vi "LVClass_Pupil ctor from dimensions.vi"(0 "Pupil (const)":refnum<class "Pupil.lvclass">, 5 "Dimensions_um":T1, 7 "value":u8=1, 11 "error in (no error)":errorcluster) -> (4 "Pupil (new)":refnum<class "Pupil.lvclass">, 15 "error out":errorcluster)   [LabVIEW 2020, in "Pupil.lvclass"]
doc: "Pupil constructor from dimensions, steps and inital value.\n\n--------------------------------------------------------------------------------\n\n<B>PupilIn </B> : Constant Pointer to Pupil object.\n<B>PupilOut </B> : Constant Pointer to Pupil object.\n<B>dimensions </B> : Pupil array dimensions (width, height).\n<B>steps </B> : Step x and y between the subpupils (um).\n<B>value </B> : Inital value.\n<B>ErrorIn </B> : Error\n<B>ErrorOut </B> : Error\n\n--------------------------------------------------------------------------------"
uses:
  Pupil.lvclass
  Controls/General dimensions definition.ctl
  Controls/Point2D.ctl
  Controls/Point2Df.ctl
  Controls/Handle creation.ctl
  Pupil.lvclass/Pupil.ctl
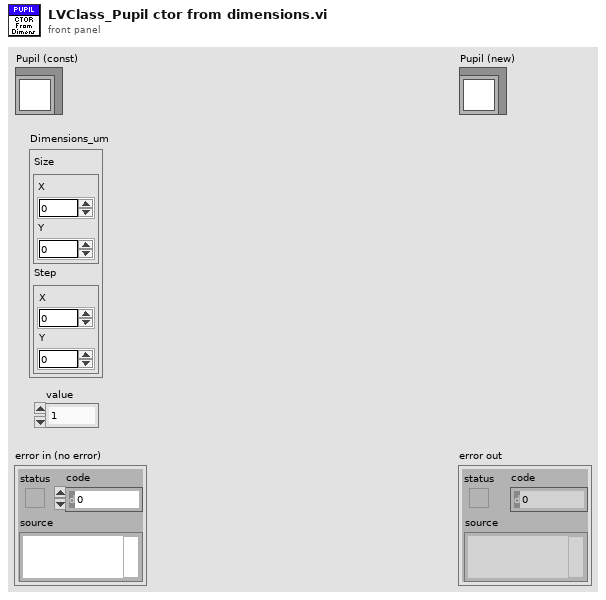
[diagram p1: front panel]
types:
  T1 = typedef "General dimensions definition.ctl" = cluster{"Size":T2, "Step":T3}
  T2 = typedef "Point2D.ctl" = cluster{"X":u32, "Y":u32}
  T3 = typedef "Point2Df.ctl" = cluster{"X":sgl, "Y":sgl}
  T4 = typedef "Handle creation.ctl" = enum16{"By ctor", "By write function"}
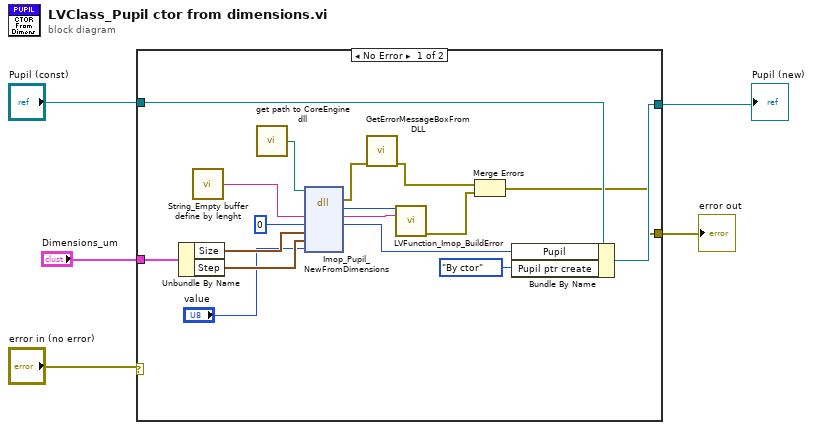
[diagram p0: block diagram]
diagram:
  n1 = case shown="No Error" "error in (no error)" {
    selector: "error in (no error)" -> [_ w23]
    tunnel: "Pupil (const)" -> [w17 w24]
    tunnel: [w18 w24] -> w3
    tunnel: [w6 w23] -> w4
    tunnel: "Dimensions_um" -> [w12 _]
    frame No Error {
      n2 = Unbundle By Name(w12) -> ("Size"=w11:T2, "Step"=w10:T3)
      n3 = call "String_Empty buffer define by lenght.vi"() -> ("Empty buffer"=w22:string)  [unwired: 1 in]
      n4 = call "get path to CoreEngine dll.vi"() -> ("path to wavekit library"=w15:path)  [unwired: 14 in, 1 out]
      n5 = dll-call lib="D:/SOFTware/CoreEngine4_Suite/SVN_trunk/LV2011_interface/DLLs/c_interface_vc100.dll" fn="Imop_Pupil_NewFromDimensions"(path in=w15, "message"=w22, "objet"=0, "dimension"=w11, "steps"=w10, "value"="value") -> (error out=w14:errorcluster, "return type"=w19:i32, "message"=w20:string, "objet"=w21:i64)  [unwired: 5 in, 1 out]
      n6 = call "GetErrorMessageBoxFromDLL.vi"("error IN"=w14) -> ("error OUT"=w8:errorcluster)  [unwired: 10 in]
      n7 = call "LVFunction_Imop_BuildError.vi"("code"=w19, "String to Prepend to source (\"\")"=w20) -> ("error out"=w7:errorcluster)  [unwired: 13 in]
      n8 = Merge Errors(w8, w7) -> (w6:errorcluster)
      n9 = Bundle By Name(cluster=w17, "Pupil"=w21, "Pupil ptr create"=Handle_creation."By ctor") -> (w18:refnum<class "Pupil.lvclass">)
    }
    frame Error {
    }
  }
  "error out" <- w4
  "Pupil (new)" <- w3
